vi "EvenQInt32.vi"(11 "Input":i32) -> (3 "Result":bool)   [LabVIEW 2013]
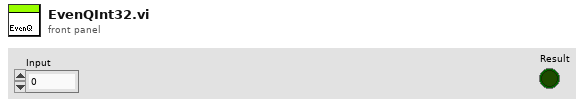
[diagram p1: front panel]
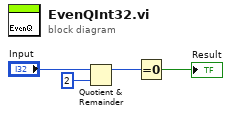
[diagram p0: block diagram]
diagram:
  n1 = Quotient & Remainder(x="Input", y=2) -> (x-y*floor(x/y)=w2:i32)  [unwired: 1 out]
  n2 = Equal To 0?(x=w2) -> (x = 0?=→"Result":bool)
